vi "仪器参数发送 (子VI).vi"(8 "错误输入":errorcluster caption="错误输出") -> (0 "错误输出":errorcluster)   [LabVIEW 2016, in "数据传输系统-04.lvlib"]
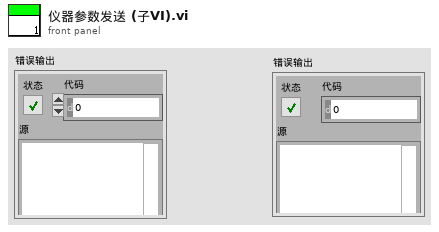
[diagram p1: front panel]
types:
  T1 = cluster{"氨氮仪器参数索引起始时间":string, "总磷仪器参数索引起始时间":string, "总氮仪器参数索引起始时间":string, "CODMn仪器参数索引起始时间":string, "CODCr仪器参数索引起始时间":string, "DO仪器参数索引起始时间":string, "PH仪器参数索引起始时间":string, "比电导率仪器参数索引起始时间":string, "水温仪器参数索引起始时间":string, "浊度仪器参数索引起始时间":string, "叶绿素a仪器参数索引起始时间":string, "藻密度仪器参数索引起始时间":string, "ORP仪器参数索引起始时间":string}
  T2 = cluster{"[0]":string, "[1]":string, "[2]":string, "[3]":string, "[4]":string, "[5]":string, "[6]":string, "[7]":string, "[8]":string, "[9]":string, "[10]":string, "[11]":string, "[12]":string}
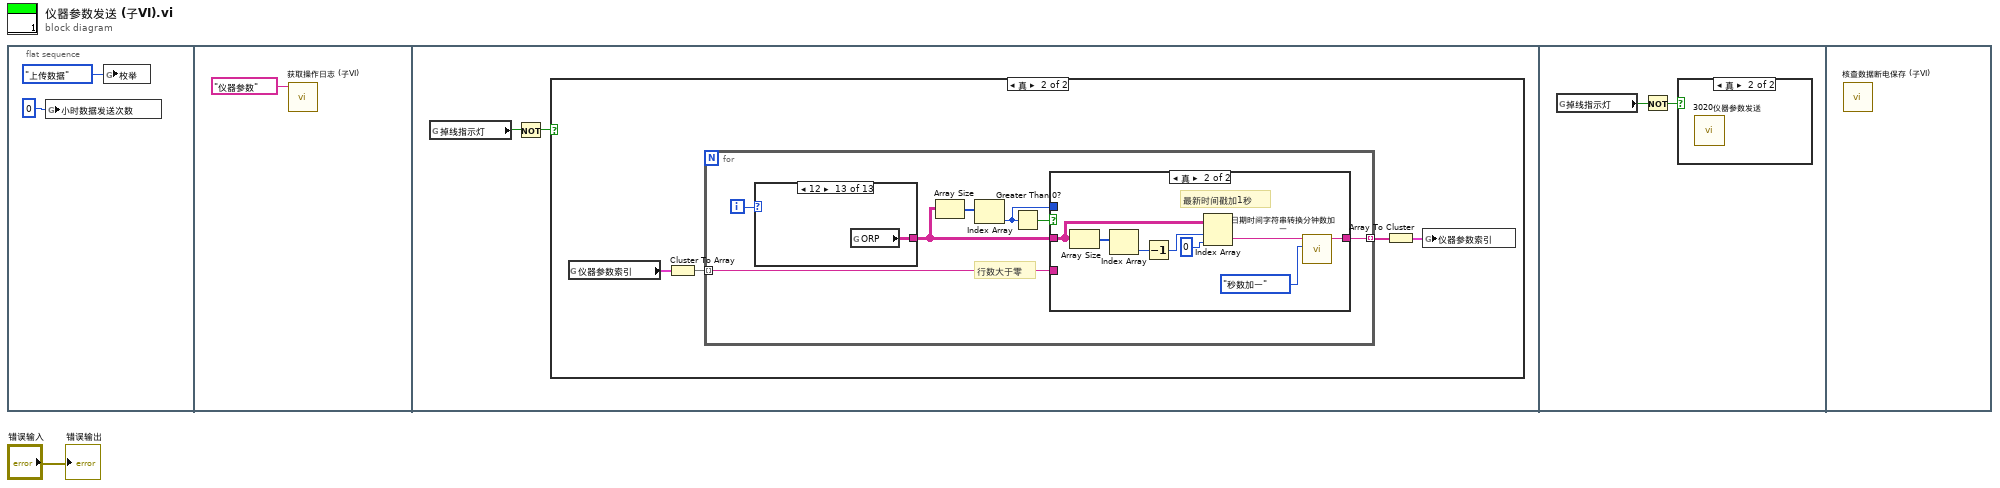
[diagram p0: block diagram]
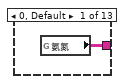
[diagram p3: hidden frame]
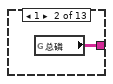
[diagram p4: hidden frame]
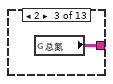
[diagram p5: hidden frame]
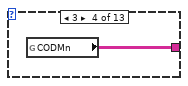
[diagram p6: hidden frame]
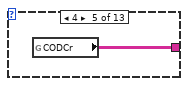
[diagram p7: hidden frame]
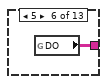
[diagram p8: hidden frame]
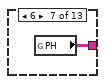
[diagram p9: hidden frame]
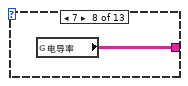
[diagram p10: hidden frame]
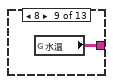
[diagram p11: hidden frame]
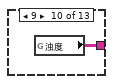
[diagram p12: hidden frame]
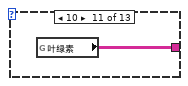
[diagram p13: hidden frame]
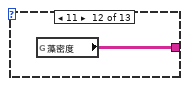
[diagram p14: hidden frame]
diagram:
  n1 = flat-sequence {
    frame #0 {
      n2 = global write "全局 小时数据发送次数.vi" "小时数据发送次数"(0 ("小时数据发送次数")) -> ()
      n3 = global write "全局1.vi" "枚举"(enum16{"返回请求应答", "上传数据", "返回执行结果"}."上传数据" ("枚举")) -> ()
    }
    frame #1 {
      n4 = call "获取操作日志 (子VI).vi"("table输入"="仪器参数") -> ()  [unwired: 11 in]
    }
    frame #2 {
      n5 = global read "全局 数据发送重叠.vi" "掉线指示灯"() -> (w6:bool)
      n6 = Not(x=w6) -> (.not. x?=w5:bool)
      n7 = case shown="真" w5 {
        frame False {
        }
        frame True {
          n8 = global read "全局 时间2.vi" "仪器参数索引"() -> (w10:T1)
          n9 = Cluster To Array(cluster=w10) -> (array=w9:string[])
          n10 = for {
            tunnel: [w14] -> w7 mode=indexing
            tunnel: w9 -> [w13] mode=indexing
            i -> [w12]
            # "行数大于零"
            n11 = case shown="12" w12 {
              tunnel: [w18 w19 w20 w21 w22 w23 w24 w25 w26 w27 w28 w29 w30] -> w11
              frame 0, Default {
                n12 = global read "全局 所有参数.vi" "氨氮"() -> (w18:string[][])
              }
              frame 1 {
                n13 = global read "全局 所有参数.vi" "总磷"() -> (w19:string[][])
              }
              frame 2 {
                n14 = global read "全局 所有参数.vi" "总氮"() -> (w20:string[][])
              }
              frame 3 {
                n15 = global read "全局 所有参数.vi" "CODMn"() -> (w21:string[][])
              }
              frame 4 {
                n16 = global read "全局 所有参数.vi" "CODCr"() -> (w22:string[][])
              }
              frame 5 {
                n17 = global read "全局 所有参数.vi" "DO"() -> (w23:string[][])
              }
              frame 6 {
                n18 = global read "全局 所有参数.vi" "PH"() -> (w24:string[][])
              }
              frame 7 {
                n19 = global read "全局 所有参数.vi" "电导率"() -> (w25:string[][])
              }
              frame 8 {
                n20 = global read "全局 所有参数.vi" "水温"() -> (w26:string[][])
              }
              frame 9 {
                n21 = global read "全局 所有参数.vi" "浊度"() -> (w27:string[][])
              }
              frame 10 {
                n22 = global read "全局 所有参数.vi" "叶绿素"() -> (w28:string[][])
              }
              frame 11 {
                n23 = global read "全局 所有参数.vi" "藻密度"() -> (w29:string[][])
              }
              frame 12 {
                n24 = global read "全局 所有参数.vi" "ORP"() -> (w30:string[][])
              }
            }
            n25 = Array Size(array=w11) -> (size(s)=w16:i32[])
            n26 = Index Array(array=w16) -> (element=w15:i32)  [unwired: 1 in]
            n27 = Greater Than 0?(x=w15) -> (x > 0?=w17:bool)
            n28 = case shown="真" w17 {
              tunnel: w15 -> [_ _]
              tunnel: w11 -> [_ w36]
              tunnel: [w31 w33] -> w14
              tunnel: w13 -> [w31 _]
              frame False {
              }
              frame True {
                # "最新时间戳加1秒"
                n29 = Array Size(array=w36) -> (size(s)=w38:i32[])
                n30 = Index Array(array=w38) -> (element=w37:i32)  [unwired: 1 in]
                n31 = Decrement(x=w37) -> (x-1=w35:i32)
                n32 = Index Array(array=w36, index (row)=w35, index (col)=0 ("禁用的索引 (列)")) -> (element=w39:string)
                n33 = call "日期时间字符串转换分钟数加一.vi"("枚举"=enum16{"分钟数加一", "秒数加一", "小时数加一"}."秒数加一", "data[0]"=w39) -> ("日期/时间字符串"=w33:string)  [unwired: 9 in]
              }
            }
          }
          n34 = Array To Cluster(array=w7) -> (cluster=w8:T2)
          n35 = global write "全局 时间2.vi" "仪器参数索引"(w8) -> ()
        }
      }
    }
    frame #3 {
      n36 = global read "全局 数据发送重叠.vi" "掉线指示灯"() -> (w41:bool)
      n37 = Not(x=w41) -> (.not. x?=w40:bool)
      n38 = case shown="真" w40 {
        frame False {
        }
        frame True {
          n39 = call "3020仪器参数发送.vi"() -> ()  [unwired: 12 in]
        }
      }
    }
    frame #4 {
      n40 = call "核查数据断电保存 (子VI).vi"() -> ()  [unwired: 12 in]
    }
  }
  "错误输出" <- "错误输入"
